vi "Pre Launch Init.vi"(11 "HL7 in":refnum<class "HL7.lvclass"> caption="操作者输入") -> (0 "error out":errorcluster caption="错误输出", 3 "HL7 out":refnum<class "HL7.lvclass"> caption="操作者输出")   [LabVIEW 2016, in "HL7.lvlib" / "HL7.lvclass"]
doc: "(<B>Filename</B>: Actor Framework.lvlib:Actor.lvclass:Pre Launch Init.vi)\n\nDefines behavior that occurs after the Launch Nested Actor method is invoked but before the actor's Actor Core method begins running.\n\nBy default, this method does nothing.子孙类重写该方法定义具体的操作。"
uses:
  HL7.lvclass
  <vilib>/ActorFramework/Actor/Actor.lvclass
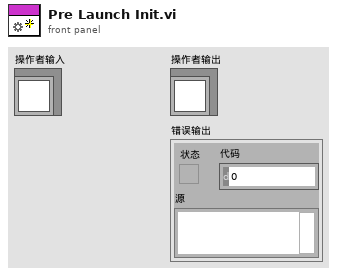
[diagram p1: front panel]
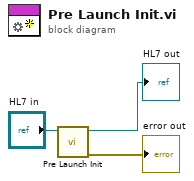
[diagram p0: block diagram]
diagram:
  n1 = call-parent "Pre Launch Init.vi"("Actor in"="HL7 in") -> ("error out"=→"error out":errorcluster, "Actor out"=→"HL7 out":refnum<class "HL7.lvclass">)  [unwired: 9 in]
